vi "Try Update Config.vi"(8 "error in (no error)":errorcluster, 11 "Volatus Core in":refnum<class "Volatus Core.lvclass">) -> (0 "error out":errorcluster, 3 "Volatus Core out":refnum<class "Volatus Core.lvclass">)   [LabVIEW 2020, in "Volatus.lvlib" / "Volatus Core.lvclass"]
uses:
  Volatus Core.lvclass
  C:/dev/lv20CE/relink/lv-volatus/Volatus/Module/Module.lvclass
  Config Updater/Config Updater.lvclass
  Volatus Core.lvclass/Volatus Core.ctl
  Module/Module.lvclass/Module.ctl
  Module/Module.lvclass
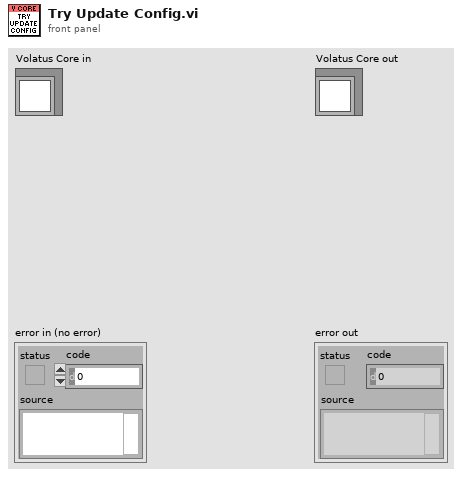
[diagram p1: front panel]
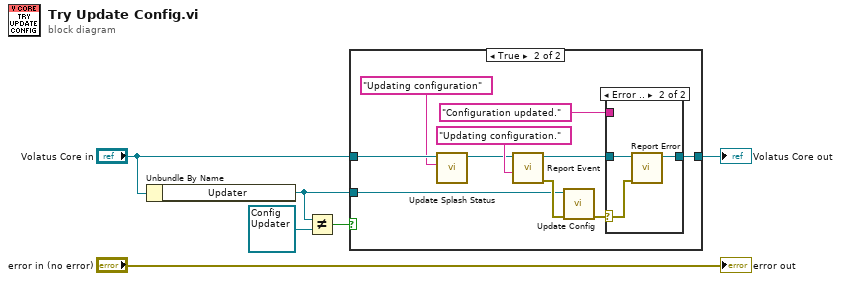
[diagram p0: block diagram]
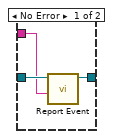
[diagram p3: hidden frame]
diagram:
  n1 = Unbundle By Name("Volatus Core in") -> ("Updater"=w3:refnum<class "Config Updater.lvclass">)
  n2 = Not Equal?(x=w3, y=refnum<class "Config Updater.lvclass"> refnum) -> (x != y?=w4:bool)
  n3 = case shown="True" w4 {
    tunnel: w3 -> [_ w15]
    tunnel: "Volatus Core in" -> [w7 w14]
    tunnel: [w7 w10] -> w1
    frame False {
      # "Updater not specified."
    }
    frame True {
      n4 = call "Update Splash Status.vi"("Status"="Updating configuration", "Volatus Core in"=w14) -> ("Volatus Core out"=w9:refnum<class "Volatus Core.lvclass">)  [unwired: 8 in, 1 out]
      n5 = call "Report Event.vi"("Message"="Updating configuration.", "Module in"=w9) -> ("error out"=w17:errorcluster, "Module out"=w12:refnum<class "Volatus Core.lvclass">)  [unwired: 8 in]
      n6 = call-dynamic "Update Config.vi"("error in (no error)"=w17, "Config Updater in"=w15) -> ("error out"=w13:errorcluster)  [unwired: 9 in]
      n7 = case shown="Error .." w13 {
        selector: w13 -> [_ w22]
        tunnel: w12 -> [w20 w23]
        tunnel: "Configuration updated." ("Message") -> [w19 _]
        tunnel: [w18 w21] -> w10
        frame No Error {
          n8 = call "Report Event.vi"("Message"=w19, "Module in"=w20) -> ("Module out"=w18:refnum<class "Volatus Core.lvclass">)  [unwired: 8 in, 1 out]
        }
        frame Error {
          n9 = call "Report Error.vi"("error in (no error)"=w22, "Module in"=w23) -> ("Module out"=w21:refnum<class "Volatus Core.lvclass">)  [unwired: 8 in, 1 out]
        }
      }
    }
  }
  "Volatus Core out" <- w1
  "error out" <- "error in (no error)"
